vi "Log Field.vi"(8 "error in (no error)":errorcluster, 11 "Power Supply In":refnum<class "Power Supply.lvclass">) -> (0 "error out":errorcluster, 3 "Power Supply Out":refnum<class "Power Supply.lvclass">)   [LabVIEW 2009, in "Power Supply.lvclass"]
uses:
  Power Supply.lvclass
  Power Supply.lvclass/Power Supply.ctl
  Global/File Locations.vi
panel:
  out "Field":dbl[unit]
  out "status":string
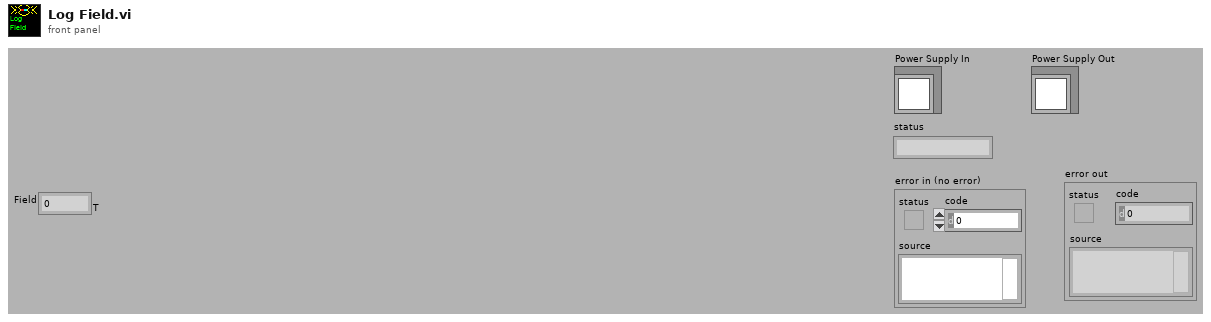
[diagram p1: front panel]
types:
  T1 = enum16{"open", "open or create", "create or replace", "create", "open (read only)"}
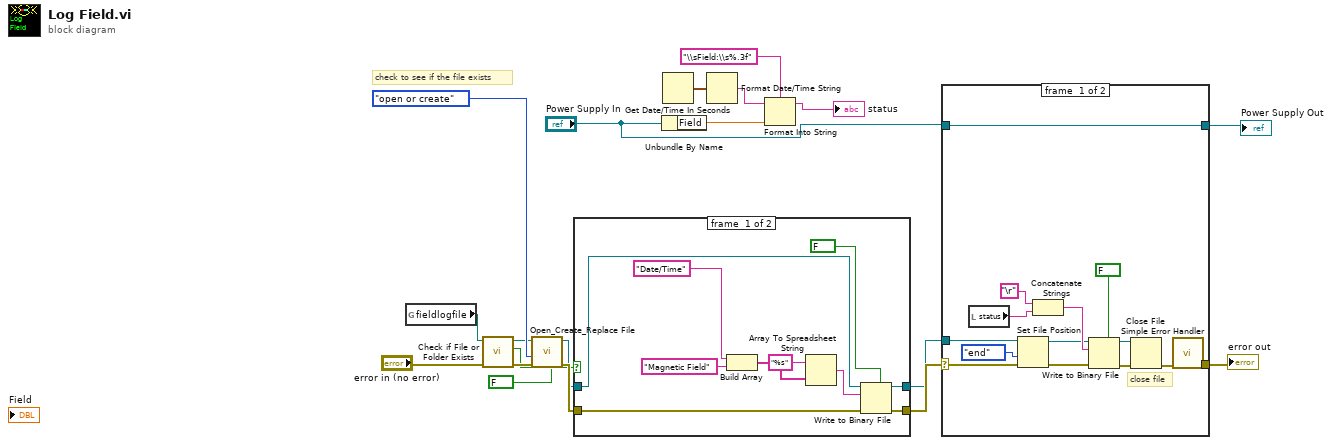
[diagram p0: block diagram]
diagram:
  # "check to see if the file exists"
  n1 = global read "File Locations.vi" "fieldlogfile"() -> (w10:path)
  n2 = call <vilib>:"Check if File or Folder Exists.vi"("error in (no error)"="error in (no error)", "path"=w10) -> ("error out"=w18:errorcluster, "file or folder exists?"=w14:bool, "dup path"=w15:path)  [unwired: 7 out]
  n3 = call <vilib>:"Open_Create_Replace File.vi"("advisory dialog? (display:T)"=FALSE, "error in (no error)"=w18, "function (open:0)"=T1."open or create", "file path"=w15) -> ("error out"=w17:errorcluster, "refnum"=w16:refnum<file>)  [unwired: 3 in, 3 out]
  n4 = case shown="False" w14 {
    tunnel: w16 -> [w29 w31]
    tunnel: w17 -> [w28 w30]
    tunnel: [w26 w31] -> w11
    tunnel: [w25 w30] -> w12
    frame #0 {
      n5 = Build Array("Date/Time", "Magnetic Field" ("element")) -> (w22:string[])
      n6 = Array To Spreadsheet String(array=w22, 3:"%s" ("format string")) -> (spreadsheet string=w21:string)  [unwired: 1 in]
      n7 = Write to Binary File(file (use dialog)=w29, data=w21, error in=w28, 5:FALSE ("prepend array or string size? (T)")) -> (refnum out=w26:refnum<file>, error out=w25:errorcluster)  [unwired: 3 out]
    }
    frame #1 {
    }
  }
  n8 = Unbundle By Name("Power Supply In") -> ("Field"=w3:dbl[unit])
  n9 = Get Date/Time In Seconds() -> (seconds since 1Jan1904=w4:timestamp)
  n10 = Format Date/Time String(seconds (now)=w4) -> (date/time string=w5:string)  [unwired: 2 in]
  n11 = Format Into String(format string="\\sField:\\s%.3f", initial string=w5, w3) -> (resulting string=→"status":string)  [unwired: 1 in, 1 out]
  n12 = case shown="No Error" w12 {
    selector: w12 -> [w39 w47]
    tunnel: w11 -> [w44 _]
    tunnel: [w40 w47] -> w9
    tunnel: "Power Supply In" -> [w32 w46]
    tunnel: [w32 w46] -> w7
    frame #0 {
      # "close file"
      n13 = local read "status"() -> (w36:string)
      n14 = Set File Position(refnum=w44, from (0:start)=enum16{"start", "end", "current"}."end", error in=w39) -> (refnum out=w34:refnum<file>, error out=w33:errorcluster)  [unwired: 1 out]
      n15 = Concatenate Strings("\r", w36) -> (w35:string)
      n16 = Write to Binary File(file (use dialog)=w34, data=w35, error in=w33, 5:FALSE ("prepend array or string size? (T)")) -> (refnum out=w45:refnum<file>, error out=w43:errorcluster)  [unwired: 3 out]
      n17 = Close File(refnum=w45, error in=w43) -> (error out=w42:errorcluster)  [unwired: 1 out]
      n18 = call <vilib>:"Simple Error Handler.vi"("error in (no error)"=w42) -> ("error out"=w40:errorcluster)  [unwired: 4 in, 4 out]
    }
    frame #1 {
    }
  }
  "Power Supply Out" <- w7
  "error out" <- w9
